vi "FTW-Ether-CreateEphemeralPair.vi"(5 "Requested Ephemeral Address":string, 11 "error in":errorcluster) -> (4 "Ephemeral Endpoint":refnum<class "FTW-Endpoint.lvclass">, 6 "Actual Ephemeral Address":string, 15 "error out":errorcluster)   [LabVIEW 2013, in "FTW-Ether.lvclass"]
uses:
  FTW-Ether.lvclass
  Endpoint/FTW-Endpoint.lvclass
  FTW-Ether-EndpointType.ctl
panel:
  # "Inputs"
  # "Outputs"
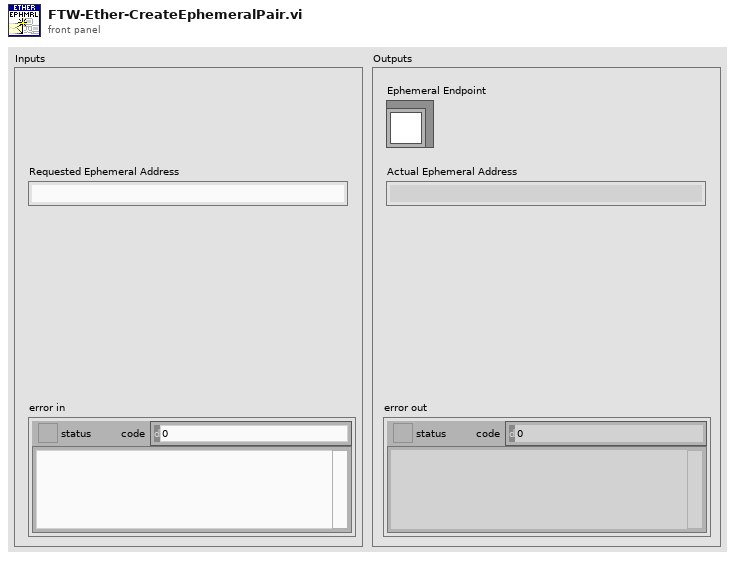
[diagram p1: front panel]
types:
  T1 = typedef "FTW-Ether.lvclass/FTW-Ether-EndpointType.ctl" = enum16{"Server", "Client", "Publisher", "Subscriber"}
  T2 = typedef "FTW-Ether.lvclass/FTW-Ether-MessageTransportScheme.ctl" = enum16{"In process (inproc://)", "TCP (tcp://)"}
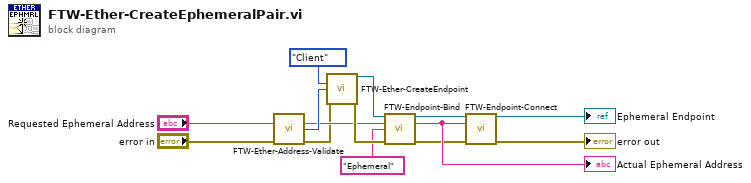
[diagram p0: block diagram]
diagram:
  n1 = call "FTW-Ether-Address-Validate.vi"("Address"="Requested Ephemeral Address", "error in"="error in") -> ("Sanitized Address"=w3:string, "Message Transport Scheme"=w4:T2, "error out"=w2:errorcluster)  [unwired: 11 in]
  n2 = call "FTW-Ether-CreateEndpoint.vi"("Endpoint Type"=FTW-Ether-EndpointType."Client", "Message Transport Scheme"=w4, "error in"=w2) -> ("FTW Endpoint"=w8:refnum<class "FTW-Endpoint.lvclass">, "error out"=w6:errorcluster)  [unwired: 11 in]
  n3 = call-dynamic "FTW-Endpoint-Bind.vi"("FTW Endpoint"=w8, "Endpoint Address"=w3, "Requested Identity"="Ephemeral", "error in"=w6) -> ("FTW Endpoint out"=w7:refnum<class "FTW-Endpoint.lvclass">, "Actual Endpoint Address"=w13:string, "error out"=w5:errorcluster)  [unwired: 8 in, 1 out]
  "Actual Ephemeral Address" <- w13
  n4 = call-dynamic "FTW-Endpoint-Connect.vi"("FTW Endpoint"=w7, "Endpoint Address"=w13, "error in"=w5) -> ("FTW Endpoint out"=→"Ephemeral Endpoint":refnum<class "FTW-Endpoint.lvclass">, "error out"=→"error out":errorcluster)  [unwired: 11 in]
